vi "FTW-Request-Reply.vi"(0 "FTW Incoming Request":refnum<class "FTW-Request.lvclass">, 11 "error in":errorcluster) -> (6 "Timed out?":bool, 15 "error out":errorcluster)   [LabVIEW 2013, in "FTW-Actor.lvlib" / "FTW-Request.lvclass"]
uses:
  FTW-Request.lvclass
  FTW-Request.lvclass/FTW-Request.ctl
  Core/src/JSON/FTW-JSON.lvclass
panel:
  # "Inputs"
  # "Outputs"
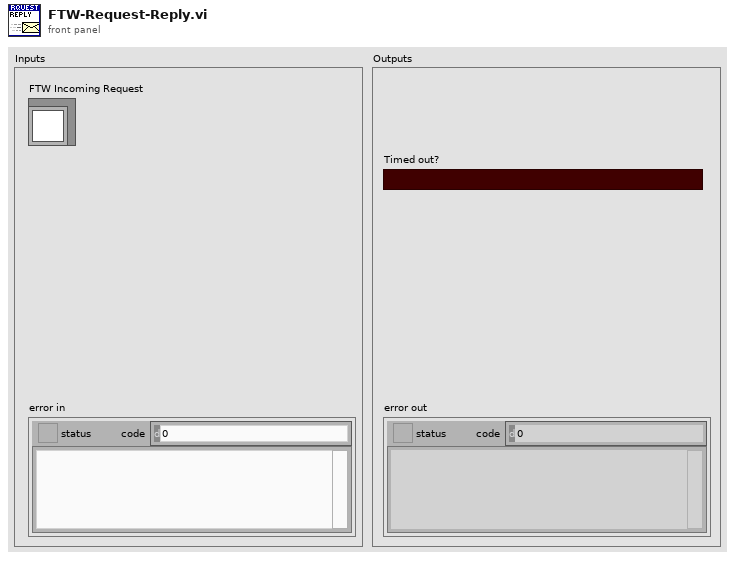
[diagram p1: front panel]
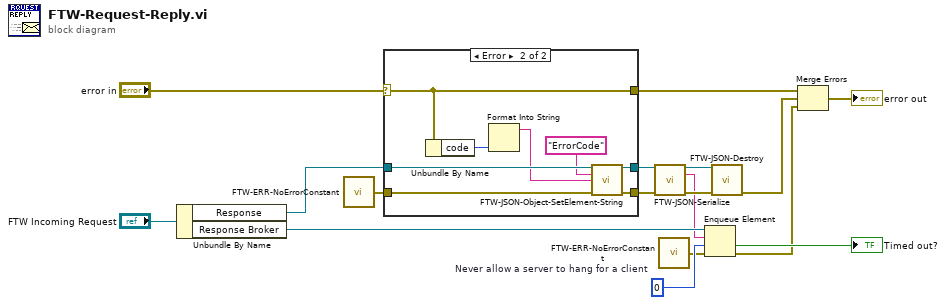
[diagram p0: block diagram]
diagram:
  w15 = 0  # Never allow a server to hang for a client
  n1 = Unbundle By Name("FTW Incoming Request") -> ("Response"=w7:refnum<class "FTW-JSON.lvclass">, "Response Broker"=w16:refnum<queue>)
  n2 = call "FTW-ERR-NoErrorConstant.vi"() -> ("no error"=w2:errorcluster)
  n3 = case shown="Error" "error in" {
    selector: "error in" -> [w19 w23]
    tunnel: w7 -> [w20 w28]
    tunnel: [w20 w27] -> w6
    tunnel: [w19 w23] -> w4
    tunnel: [w18 w25] -> w3
    tunnel: w2 -> [w18 w24]
    frame No Error {
    }
    frame Error {
      n4 = Unbundle By Name(w23) -> ("code"=w22:i32)
      n5 = Format Into String(w22) -> (resulting string=w21:string)  [unwired: 3 in, 1 out]
      n6 = call "FTW-JSON-Object-SetElement-String.vi"("JSON Object"=w28, "Key"="ErrorCode", "Value"=w21, "error in"=w24) -> ("JSON Object out"=w27:refnum<class "FTW-JSON.lvclass">, "error out"=w25:errorcluster)  [unwired: 10 in]
    }
  }
  n7 = call "FTW-JSON-Serialize.vi"("JSON Object"=w6, "error in"=w3) -> ("JSON Object out"=w13:refnum<class "FTW-JSON.lvclass">, "JSON String (UTF-8)"=w11:string, "error out"=w12:errorcluster)  [unwired: 11 in]
  n8 = call "FTW-ERR-NoErrorConstant.vi"() -> ("no error"=w1:errorcluster)
  n9 = Enqueue Element(queue=w16, element=w11, timeout in ms (-1)=w15, error in (no error)=w1) -> (timed out?=→"Timed out?":bool, error out=w9:errorcluster)  [unwired: 1 out]
  n10 = call "FTW-JSON-Destroy.vi"("JSON Object"=w13, "error in"=w12) -> ("error out"=w10:errorcluster)  [unwired: 13 in]
  n11 = Merge Errors(w4, w10, w9) -> (→"error out":errorcluster)
